vi "createCommandList.vi"(8 "error in (no error)":errorcluster, 10 "Parameters":u32[](array[numeric]), 11 "ESD in":refnum<class "ESD.lvclass">) -> (0 "error out":errorcluster, 2 "Commandlist":string, 3 "ESD out":refnum<class "ESD.lvclass">)   [LabVIEW 2013, in "ESD.lvclass"]
uses:
  ESD.lvclass
  TestInterface/TestInterface.lvclass
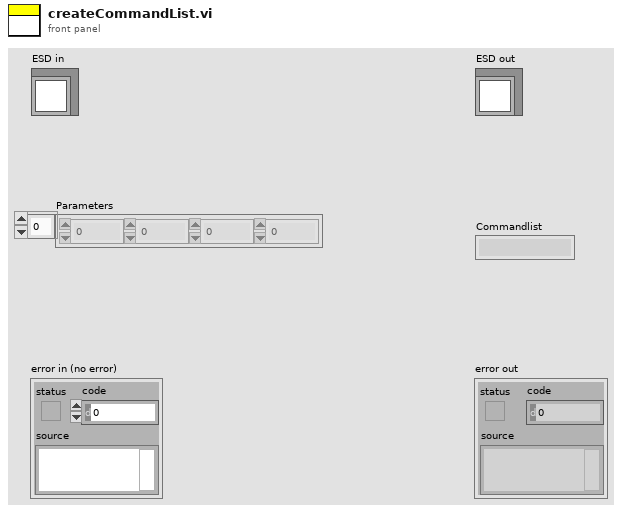
[diagram p1: front panel]
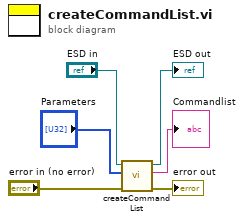
[diagram p0: block diagram]
diagram:
  n1 = call-parent "createCommandList.vi"("error in (no error)"="error in (no error)", "Parameters"="Parameters", "TestInterface in"="ESD in") -> ("error out"=→"error out":errorcluster, "Commandlist"=→"Commandlist":string, "TestInterface out"=→"ESD out":refnum<class "ESD.lvclass">)  [unwired: 6 in]
